vi "createTable.vi"(11 "Input board":refnum<class "Cell.lvclass">[][](array[class])=[[refnum, refnum, refnum, refnum, refnum, refnum], [refnum, refnum, refnum, refnum, refnum, refnum], [refnum, refnum, refnum, refnum, refnum, refnum], [refnum, refnum, refnum, refnum, refnum, refnum], [refnum, refnum, refnum, refnum, refnum, refnum], [refnum, refnum, refnum, refnum, refnum, refnum]]) -> (2 "Array 2":bool[][](array[boolean]), 3 "Array":picture[][](array[picture]))   [LabVIEW 2014]
uses:
  Cell.lvclass
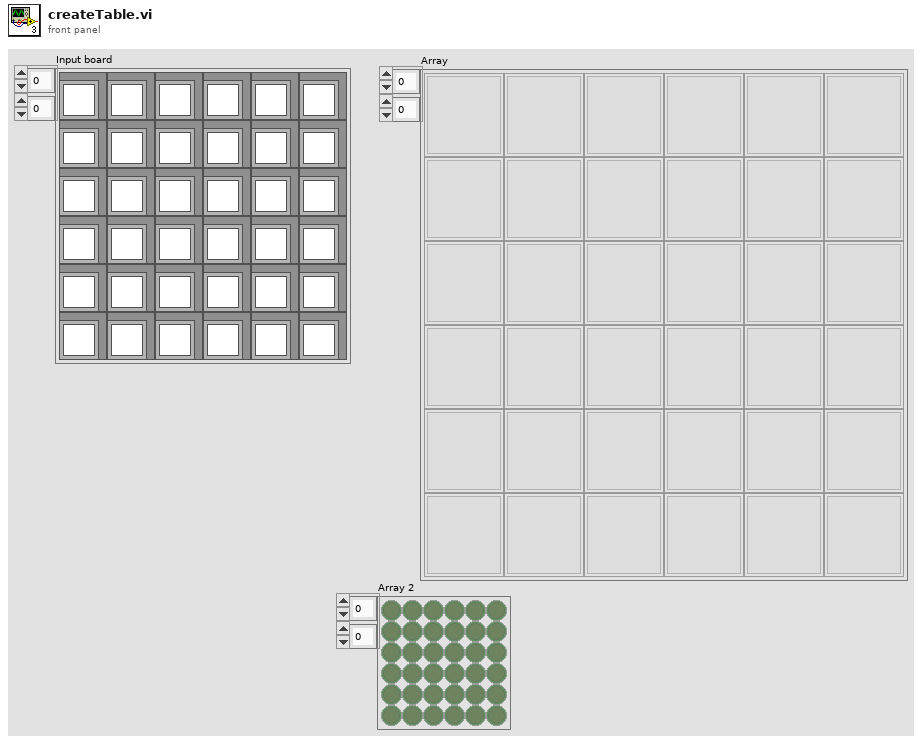
[diagram p1: front panel]
types:
  T1 = typedef "imagedata.ctl" = cluster{"image type":i32, "image depth":i32, "image":u8[], "mask":u8[], "colors":u32[], "Rectangle":cluster{"left":i16, "top":i16, "right":i16, "bottom":i16}}
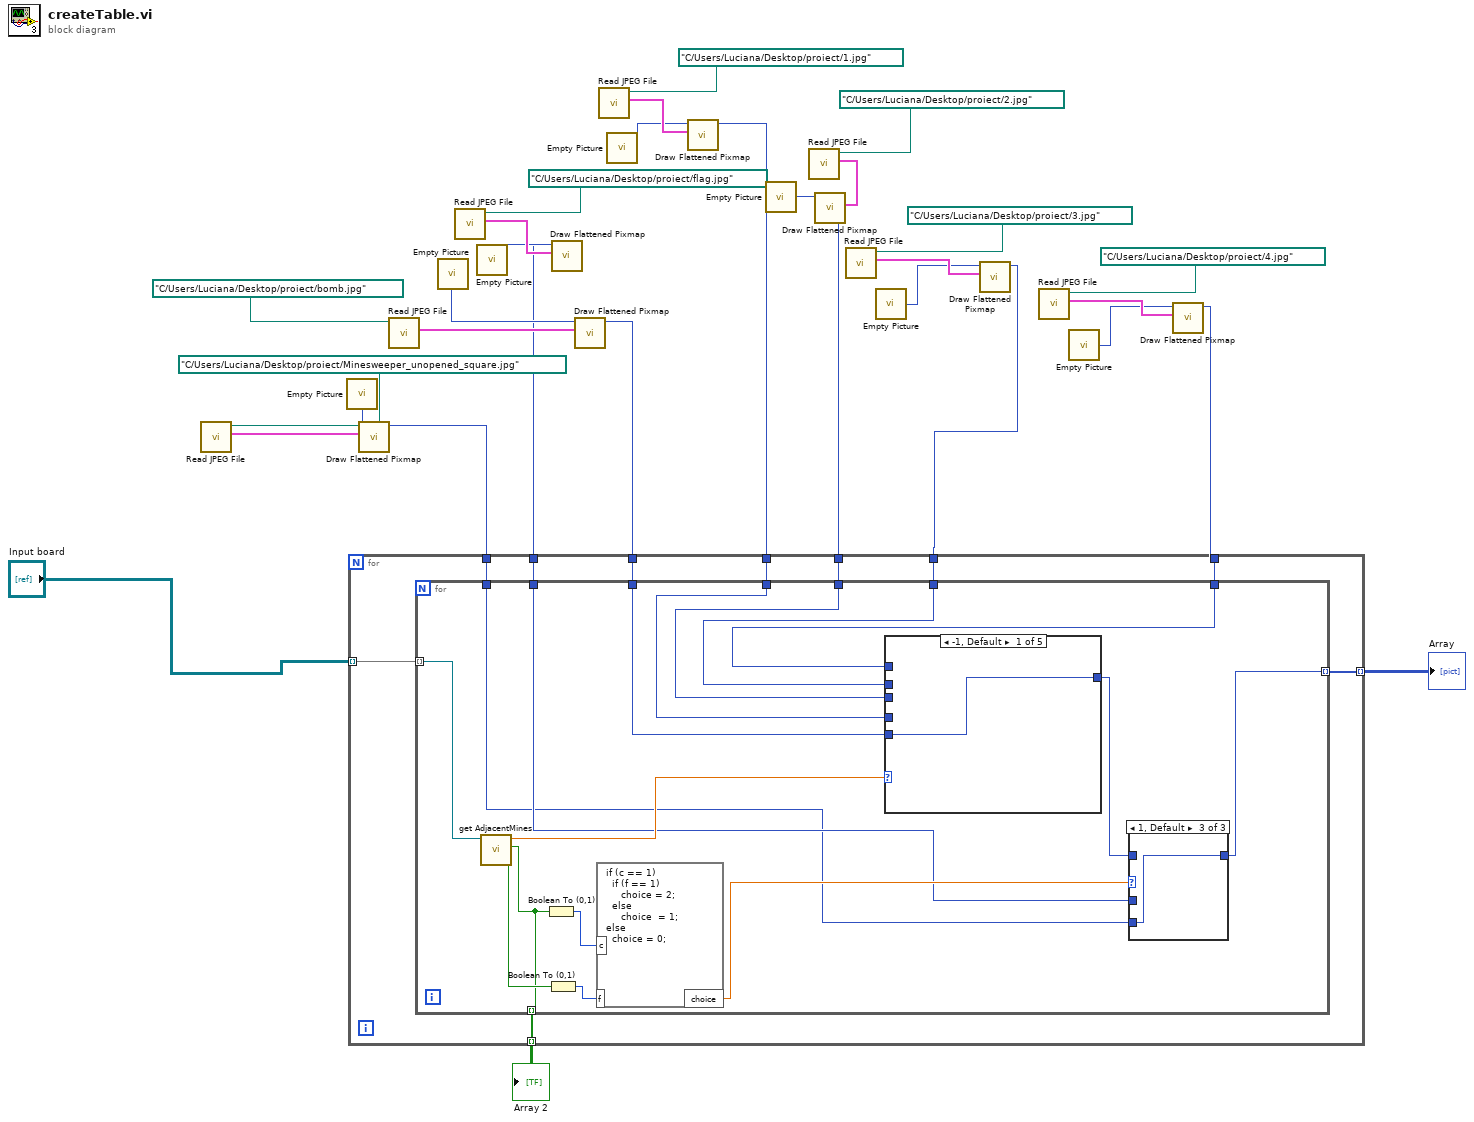
[diagram p0: block diagram]
diagram:
  n1 = call <vilib>:"Read JPEG File.vi"("path to JPEG file"=path "C:/Users/Luciana/Desktop/proiect/Minesweeper_unopened_square.jpg") -> ("image data"=w31:T1)  [unwired: 8 in, 2 out]
  n2 = call "Empty Picture"() -> ("empty picture"=w14:picture)
  n3 = call <vilib>:"Draw Flattened Pixmap.vi"("image data"=w31, "picture"=w14) -> ("new picture"=w29:picture)  [unwired: 7 in]
  n4 = call <vilib>:"Read JPEG File.vi"("path to JPEG file"=path "C:/Users/Luciana/Desktop/proiect/bomb.jpg" ("path to JPEG file 2")) -> ("image data"=w28:T1)  [unwired: 8 in, 2 out]
  n5 = call "Empty Picture"() -> ("empty picture"=w12:picture)
  n6 = call <vilib>:"Read JPEG File.vi"("path to JPEG file"=path "C:/Users/Luciana/Desktop/proiect/flag.jpg") -> ("image data"=w26:T1)  [unwired: 8 in, 2 out]
  n7 = call "Empty Picture"() -> ("empty picture"=w11:picture)
  n8 = call <vilib>:"Draw Flattened Pixmap.vi"("image data"=w26, "picture"=w11) -> ("new picture"=w10:picture)  [unwired: 7 in]
  n9 = call <vilib>:"Draw Flattened Pixmap.vi"("image data"=w28, "picture"=w12) -> ("new picture"=w13:picture)  [unwired: 7 in]
  n10 = call <vilib>:"Read JPEG File.vi"("path to JPEG file"=path "C:/Users/Luciana/Desktop/proiect/1.jpg") -> ("image data"=w24:T1)  [unwired: 8 in, 2 out]
  n11 = call "Empty Picture"() -> ("empty picture"=w9:picture)
  n12 = call <vilib>:"Draw Flattened Pixmap.vi"("image data"=w24, "picture"=w9) -> ("new picture"=w22:picture)  [unwired: 7 in]
  n13 = call "Empty Picture"() -> ("empty picture"=w8:picture)
  n14 = call <vilib>:"Read JPEG File.vi"("path to JPEG file"=path "C:/Users/Luciana/Desktop/proiect/2.jpg") -> ("image data"=w21:T1)  [unwired: 8 in, 2 out]
  n15 = call <vilib>:"Draw Flattened Pixmap.vi"("image data"=w21, "picture"=w8) -> ("new picture"=w19:picture)  [unwired: 7 in]
  n16 = call <vilib>:"Read JPEG File.vi"("path to JPEG file"=path "C:/Users/Luciana/Desktop/proiect/3.jpg") -> ("image data"=w18:T1)  [unwired: 8 in, 2 out]
  n17 = call "Empty Picture"() -> ("empty picture"=w16:picture)
  n18 = call <vilib>:"Draw Flattened Pixmap.vi"("image data"=w18, "picture"=w16) -> ("new picture"=w15:picture)  [unwired: 7 in]
  n19 = call <vilib>:"Read JPEG File.vi"("path to JPEG file"=path "C:/Users/Luciana/Desktop/proiect/4.jpg") -> ("image data"=w7:T1)  [unwired: 8 in, 2 out]
  n20 = call "Empty Picture"() -> ("empty picture"=w5:picture)
  n21 = call <vilib>:"Draw Flattened Pixmap.vi"("image data"=w7, "picture"=w5) -> ("new picture"=w4:picture)  [unwired: 7 in]
  n22 = for {
    tunnel: w29 -> [w41]
    tunnel: "Input board" -> [w40] mode=indexing
    tunnel: w13 -> [w39]
    tunnel: w10 -> [w38]
    tunnel: w22 -> [w37]
    tunnel: w19 -> [w36]
    tunnel: w15 -> [w35]
    tunnel: w4 -> [w34]
    tunnel: [w33] -> w3 mode=indexing
    tunnel: [w32] -> w1 mode=indexing
    n23 = for {
      tunnel: w41 -> [w43]
      tunnel: w40 -> [w57] mode=indexing
      tunnel: w39 -> [w55]
      tunnel: w38 -> [w44]
      tunnel: w37 -> [w54]
      tunnel: w36 -> [w53]
      tunnel: w35 -> [w52]
      tunnel: w34 -> [w47]
      tunnel: [w45] -> w33 mode=indexing
      tunnel: [w42] -> w32 mode=indexing
      n24 = call-dynamic "get AdjacentMines.vi"("Cell in"=w57) -> ("hasFlag"=w50:bool, "isCovered"=w42:bool, "AdjacentMines"=w56:dbl)  [unwired: 7 in, 1 out]
      n25 = Boolean To (0,1)(Boolean=w42) -> (0, 1=w51:i16)
      n26 = Boolean To (0,1)(Boolean=w50) -> (0, 1=w49:i16)
      n27 = formula code="if (c == 1)\n  if (f == 1)\n     choice = 2;\n  else\n     choice  = 1;\nelse\n  choice = 0;"("f"=w49, "c"=w51) -> ("choice"=w48:dbl)
      n28 = case shown="-1, Default" w56 {
        tunnel: w55 -> [w61 _ _ _ _]
        tunnel: [w61 w62 w63 w64 w65] -> w46
        tunnel: w54 -> [_ w62 _ _ _]
        tunnel: w53 -> [_ _ w63 _ _]
        tunnel: w52 -> [_ _ _ w64 _]
        tunnel: w47 -> [_ _ _ _ w65]
        frame -1, Default {
        }
        frame 1 {
        }
        frame 2 {
        }
        frame 3 {
        }
        frame 4 {
        }
      }
      n29 = case shown="1, Default" w48 {
        tunnel: w46 -> [w58 _ _]
        tunnel: [w58 w59 w60] -> w45
        tunnel: w44 -> [_ w59 _]
        tunnel: w43 -> [_ _ w60]
        frame 0 {
        }
        frame 2 {
        }
        frame 1, Default {
        }
      }
    }
  }
  "Array" <- w3
  "Array 2" <- w1
